vi "wfm_feature add_area_plot.vi"(8 "error in (no error)":errorcluster, 10 "fill graph param":T1, 11 "wfm_feature in":refnum<class "wfm_feature.lvclass">) -> (0 "error out":errorcluster, 3 "wfm_feature out":refnum<class "wfm_feature.lvclass">)   [LabVIEW 2018, in "wfm_feature.lvclass"]
uses:
  wfm_feature.lvclass
  wfm_feature.lvclass/wfm_feature.ctl
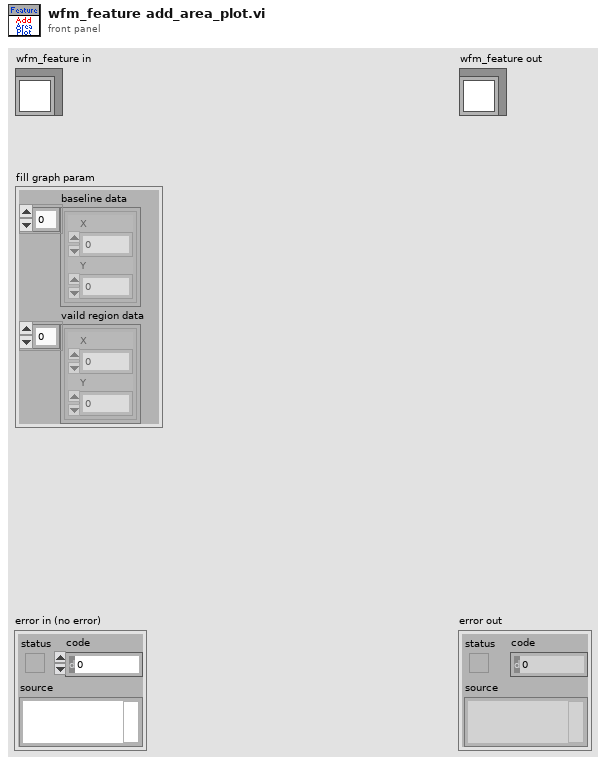
[diagram p1: front panel]
types:
  T1 = cluster{"baseline data":cluster{"X":dbl, "Y":dbl}[], "vaild region data":cluster{"X":dbl, "Y":dbl}[]}
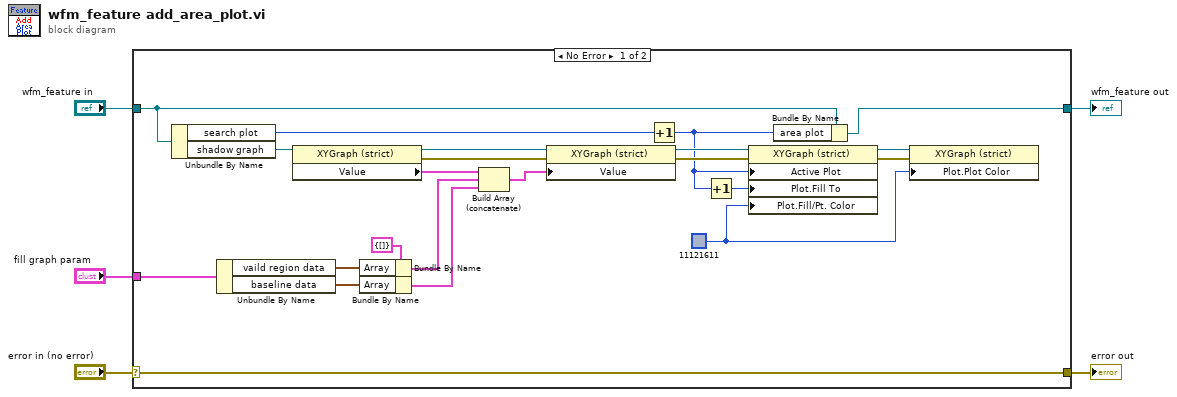
[diagram p0: block diagram]
diagram:
  n1 = case shown="No Error" "error in (no error)" {
    selector: "error in (no error)" -> [w27 w29]
    tunnel: [w27 w29] -> w4
    tunnel: [w19 w28] -> w2
    tunnel: "wfm_feature in" -> [w20 w28]
    tunnel: "fill graph param" -> [w12 _]
    frame No Error {
      w8 = u32 11121611
      w26 = cluster{"Array":cluster{"X":dbl, "Y":dbl}[]} {"Array"=[]} ("element")
      n2 = Unbundle By Name(w20) -> ("search plot"=w21:i32, "shadow graph"=w25:refnum<vi>)
      n3 = Unbundle By Name(w12) -> ("vaild region data"=w11:cluster{"X":dbl, "Y":dbl}[], "baseline data"=w10:cluster{"X":dbl, "Y":dbl}[])
      n4 = property class="XYGraph (strict)"(reference=w25) -> (reference out=w18:refnum<vi>, error out=w17:errorcluster, "Value"=w24:cluster{"Array":cluster{"X":dbl, "Y":dbl}[]}[])  [unwired: 1 in]
      n5 = Bundle By Name(cluster=w26, "Array"=w11) -> (w23:cluster{"Array":cluster{"X":dbl, "Y":dbl}[]})
      n6 = Bundle By Name(cluster=w26, "Array"=w10) -> (w22:cluster{"Array":cluster{"X":dbl, "Y":dbl}[]})
      n7 = Build Array (concatenate)(w24, w23, w22) -> (w16:cluster{"Array":cluster{"X":dbl, "Y":dbl}[]}[])
      n8 = property class="XYGraph (strict)"(reference=w18, error in=w17, "Value"=w16) -> (reference out=w15:refnum<vi>, error out=w14:errorcluster)
      n9 = Increment(x=w21) -> (x+1=w13:i32)
      n10 = Increment(x=w13) -> (x+1=w9:i32)
      n11 = property class="XYGraph (strict)"(reference=w15, error in=w14, "Active Plot"=w13, "Plot.Fill To"=w9, "Plot.Fill/Pt. Color"=w8) -> (reference out=w7:refnum<vi>, error out=w6:errorcluster)
      n12 = Bundle By Name(cluster=w20, "area plot"=w13) -> (w19:refnum<class "wfm_feature.lvclass">)
      n13 = property class="XYGraph (strict)"(reference=w7, error in=w6, "Plot.Plot Color"=w8) -> ()  [unwired: 2 out]
    }
    frame Error {
    }
  }
  "error out" <- w4
  "wfm_feature out" <- w2
